vi "LED flashing 4.vi"(0 "Arduino Resource In":T1={"VISA resource"="", "Board Type"=enum."Uno", "Connection Type"=enum."USB / Serial", "Bytes Per Packet (15)"=15}, 11 "Error In":errorcluster) -> (2 "1           2           3          4":bool[](array[boolean]), 4 "Arduino Resource Out":T1={"VISA resource"="", "Board Type"=enum."Uno", "Connection Type"=enum."USB / Serial", "Bytes Per Packet (15)"=15}, 15 "Error Out":errorcluster)   [LabVIEW 2016]
uses:
  <vilib>/LabVIEW Interface for Arduino/Type Defs/Arduino Resource.ctl
  <vilib>/LabVIEW Interface for Arduino/Type Defs/Board Type.ctl
  <vilib>/LabVIEW Interface for Arduino/LabVIEW Interface for Arduino.lvlib
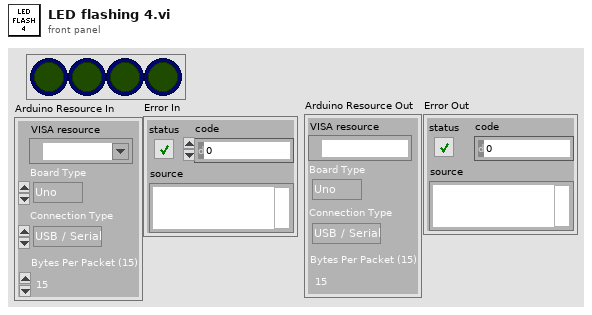
[diagram p1: front panel]
types:
  T1 = typedef "LabVIEW Interface for Arduino.lvlib/Arduino Resource.ctl" = cluster{"VISA resource":refnum<visa-resource-name>, "Board Type":T2, "Connection Type":enum8{"USB / Serial"}, "Bytes Per Packet (15)":u8}
  T2 = typedef "LabVIEW Interface for Arduino.lvlib/Board Type.ctl" = enum16{"Uno", "Dimuelanove w/Atmega 328", "Mega 2560"}
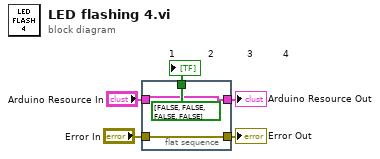
[diagram p0: block diagram]
diagram:
  n1 = flat-sequence {
    tunnel: [bool[] [FALSE, FALSE, FALSE, FALSE]] -> w5
    tunnel: [w7] -> w2
    tunnel: "Arduino Resource In" -> [w7]
    tunnel: [w6] -> w1
    tunnel: "Error In" -> [w6]
    frame #0 {
    }
  }
  "1           2           3          4" <- w5
  "Arduino Resource Out" <- w2
  "Error Out" <- w1
